vi "Gen - Get Unique Value.vi"(1 "data":string[][](array[string])) -> (0 "Unique Values":string[](array[string]))   [LabVIEW 2020]
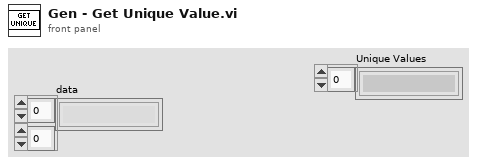
[diagram p1: front panel]
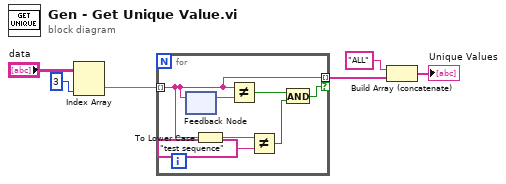
[diagram p0: block diagram]
diagram:
  n1 = Index Array(array="data", index (col)=3 ("disabled index (col)")) -> (element=w1:string[])  [unwired: 1 in]
  n2 = for {
    tunnel: w1 -> [w9] mode=indexing
    tunnel: [w9] -> w5 mode=indexing if=w11
    n3 = feedback-in #1(w9) -> ()
    n4 = feedback #1() -> (w13:string)  [unwired: 1 in]
    n5 = To Lower Case(string=w9) -> (all lower case string=w8:string)
    n6 = Not Equal?(x=w9, y=w13) -> (x != y?=w12:bool)
    n7 = Not Equal?(x=w8, y="test sequence") -> (x != y?=w10:bool)
    n8 = And(x=w12, y=w10) -> (x .and. y?=w11:bool)
  }
  n9 = Build Array (concatenate)("ALL", w5) -> (→"Unique Values":string[])
